vi "Subarray up to Step (SubVI).vi"(10 "Step Index":i32, 11 "Delay Positions":dbl[](array[numeric])) -> (3 "Array":dbl[](array[numeric]))   [LabVIEW 2020]
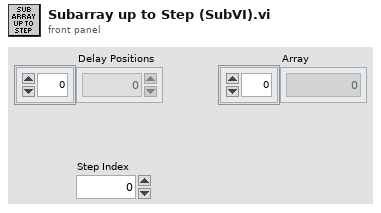
[diagram p1: front panel]
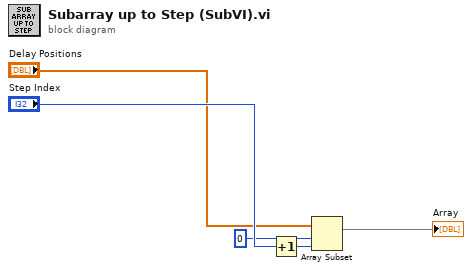
[diagram p0: block diagram]
diagram:
  n1 = Increment(x="Step Index") -> (x+1=w5:i32)
  n2 = Array Subset(array="Delay Positions", index=0, length=w5) -> (→"Array":dbl[])
